vi "data subset.vi"(1 "End time (s)":dbl, 2 "FFT interval (s)":dbl, 3 "sensor":dbl[][](array[numeric]), 4 "Frequency (Hz)":dbl) -> (0 "sensor subset":dbl[][](array[numeric]))   [LabVIEW 2009]
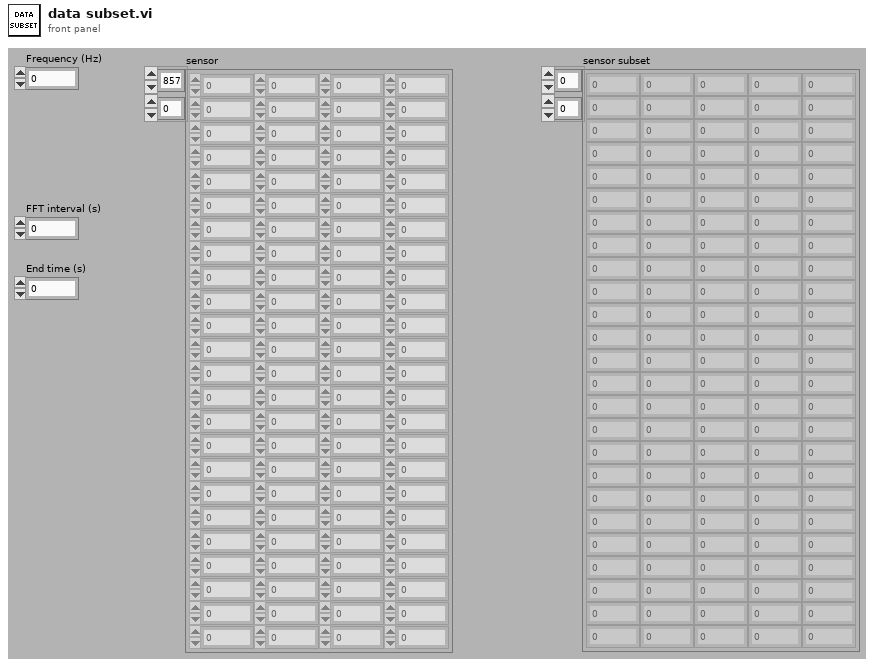
[diagram p1: front panel]
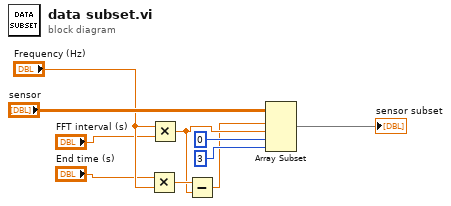
[diagram p0: block diagram]
diagram:
  n1 = Multiply(x="End time (s)", y="Frequency (Hz)") -> (x*y=w3:dbl)
  n2 = Multiply(x="Frequency (Hz)", y="FFT interval (s)") -> (x*y=w2:dbl)
  n3 = Subtract(x=w3, y=w2) -> (x-y=w1:dbl)
  n4 = Array Subset(array="sensor", index (row)=w1, length (row)=w2, index (col)=0 ("index"), length (col)=3 ("length")) -> (→"sensor subset":dbl[][])
